vi "核查数据断电保存 (子VI).vi"   [LabVIEW 2016, in "数据传输系统.lvlib"]
uses:
  <vilib>/Utility/config.llb/NI_LVConfig.lvlib
types:
  T1 = typedef "NI_LVConfig.lvlib/Config Data RefNum.ctl" = refnum<k1>
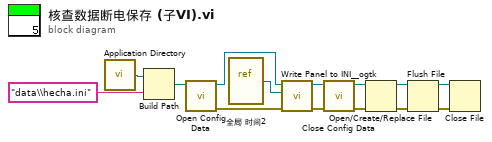
[diagram p0: block diagram]
diagram:
  n1 = call <vilib>:"Application Directory.vi"() -> ("Application Directory"=w1:path)
  n2 = Build Path(base path=w1, name or relative path="data\\hecha.ini" ("名称或相对路径")) -> (appended path=w3:path)
  n3 = call <vilib>:"Open Config Data.vi"("configuration file path"=w3) -> ("error out"=w6:errorcluster, "refnum"=w14:T1)  [unwired: 8 in, 1 out]
  n4 = vi-ref "全局 时间2.vi"() -> (w4:refnum<vi>)
  n5 = call <userlib>:"Write Panel to INI__ogtk.vi"("error in (no error)"=w6, "VI ref"=w4, "refnum"=w14) -> ("error out"=w7:errorcluster, "refnum out"=w5:T1)  [unwired: 7 in]
  n6 = call <vilib>:"Close Config Data.vi"("error in (no error)"=w7, "refnum"=w5) -> ("error out"=w12:errorcluster, "file path"=w13:path)  [unwired: 8 in]
  n7 = Open/Create/Replace File(file path (use dialog)=w13, error in=w12) -> (refnum out=w9:refnum<file>, error out=w8:errorcluster)  [unwired: 4 in, 1 out]
  n8 = Flush File(refnum=w9, error in=w8) -> (refnum out=w10:refnum<file>, error out=w11:errorcluster)
  n9 = Close File(refnum=w10, error in=w11) -> ()  [unwired: 2 out]
